vi "Handle Errors.vi"(8 "error in (no error)":errorcluster, 10 "Location":string, 11 "Mock Process In":refnum<class "Mock Process.lvclass">) -> (0 "error out":errorcluster, 3 "Mock Process Out":refnum<class "Mock Process.lvclass">)   [LabVIEW 2020, in "Mock Process.lvclass"]
doc: "The implementation of this VI defines how errors are handled."
uses:
  Mock Process.lvclass
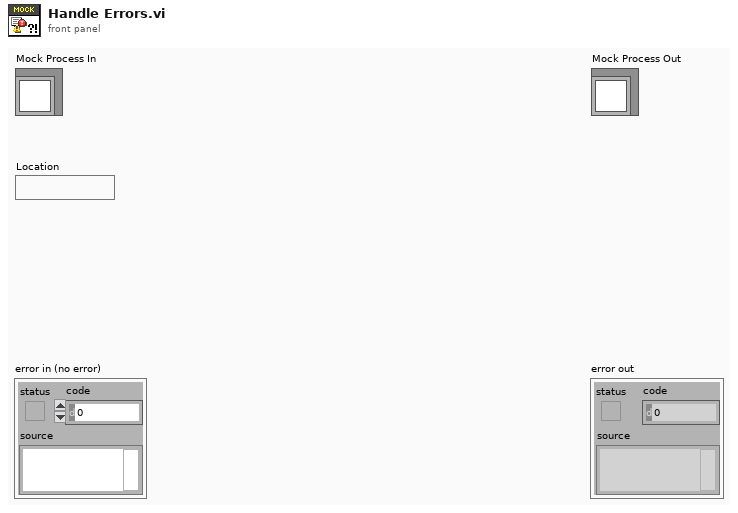
[diagram p1: front panel]
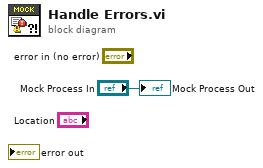
[diagram p0: block diagram]
diagram:
  "Mock Process Out" <- "Mock Process In"
